vi "closeTPDO.vi"(8 "error in (no error)":errorcluster, 10 "TPDO object in":refnum<k20>, 11 "OrionBMSClass in":refnum<class "OrionBMSClass.lvclass">) -> (0 "error in (no error) 2":errorcluster, 3 "OrionBMSClass out":refnum<class "OrionBMSClass.lvclass">)   [LabVIEW 2018, in "OrionBMSClass.lvclass"]
uses:
  OrionBMSClass.lvclass
  <vilib>/CANopenLib/CANOPEN.llb/CANopen TPDO Close.vi
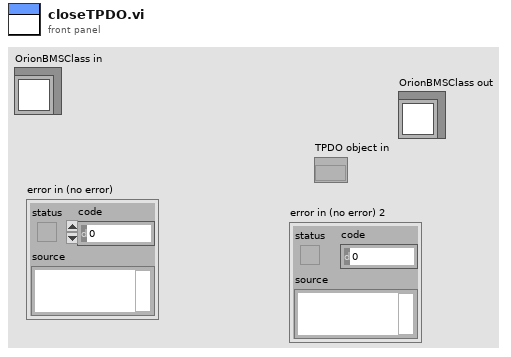
[diagram p1: front panel]
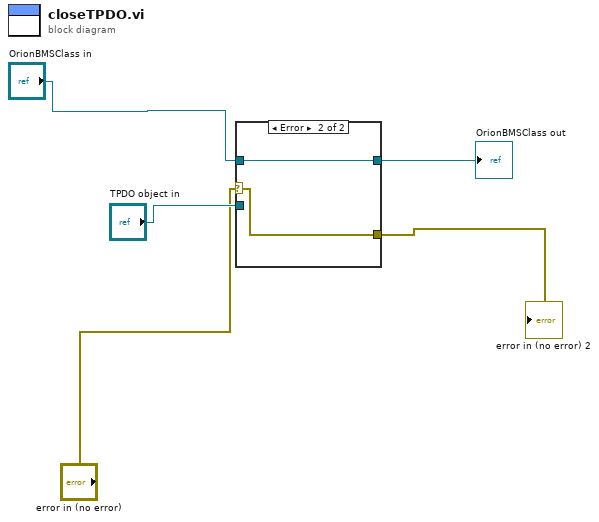
[diagram p0: block diagram]
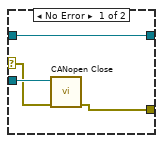
[diagram p2: hidden frame]
diagram:
  n1 = case shown="Error" "error in (no error)" {
    selector: "error in (no error)" -> [w8 w10]
    tunnel: "TPDO object in" -> [w9 _]
    tunnel: [w7 w10] -> w3
    tunnel: [w6 w11] -> w1
    tunnel: "OrionBMSClass in" -> [w6 w11]
    frame No Error {
      n2 = call-poly <vilib>:"CANopen Close.vi"("error in (no error)"=w8, "TPDO object in"=w9) -> ("error out"=w7:errorcluster)  [unwired: 9 in]
    }
    frame Error {
    }
  }
  "error in (no error) 2" <- w3
  "OrionBMSClass out" <- w1
